vi "create.vi"   [LabVIEW 2020, in "datasources.lvlib" / "source.lvclass"]
uses:
  source.lvclass
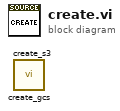
[diagram p0: block diagram]
diagram:
  n1 = call "create_gcs.vi"() -> ()  [unwired: 11 in, 1 out]
  n2 = call "create_s3.vi"() -> ()  [unwired: 11 in, 1 out]
